vi "DeMux16x16.vi"(1 "Data":bool[](array[boolean]), 2 "Select":bool[](array[boolean])) -> (0 "A":bool[][](array[boolean]))   [LabVIEW 2012]
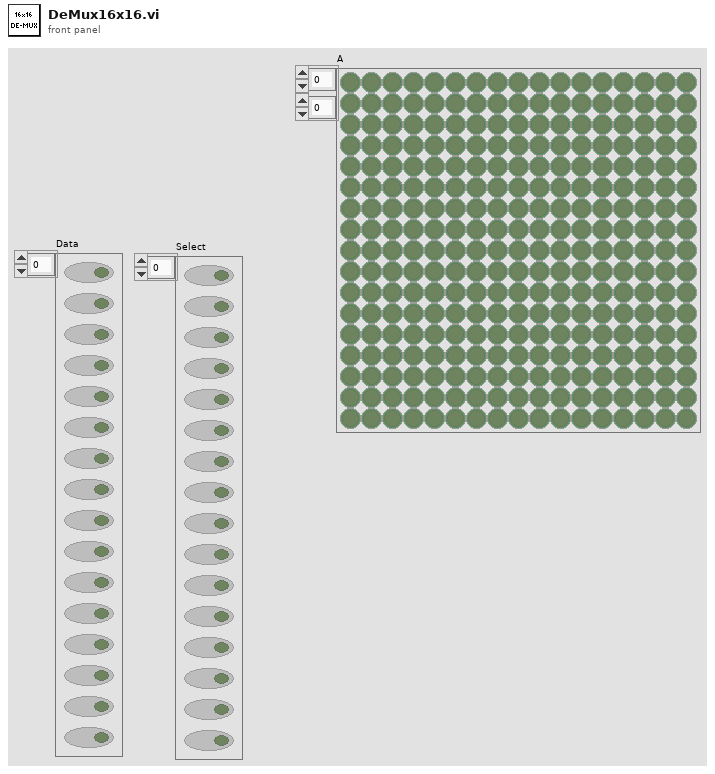
[diagram p1: front panel]
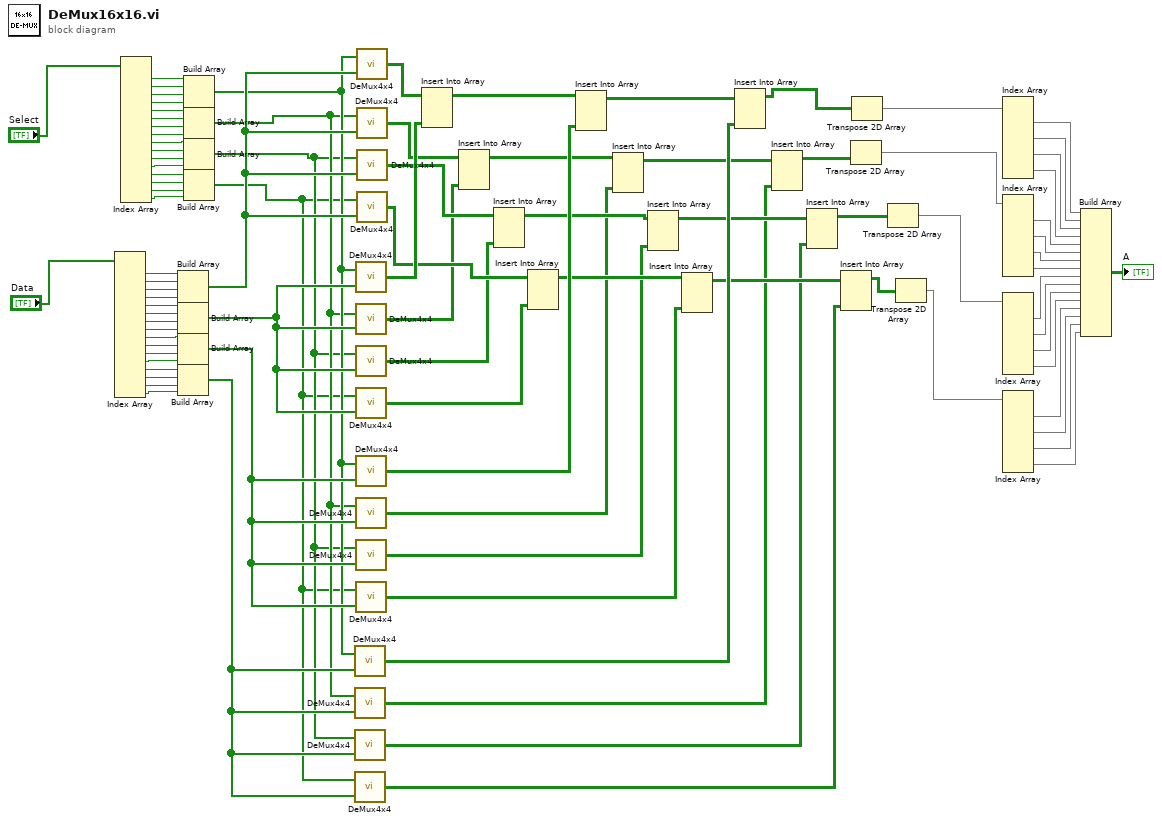
[diagram p0: block diagram]
diagram:
  n1 = Index Array(array="Data") -> (element #1=w59:bool, element #2=w60:bool, element #3=w61:bool, element #4=w62:bool, element #5=w63:bool, element #6=w64:bool, element #7=w65:bool, element #8=w66:bool, element #9=w67:bool, element #10=w68:bool, element #11=w69:bool, element #12=w70:bool, element #13=w71:bool, element #14=w72:bool, element #15=w73:bool, element #16=w74:bool)  [unwired: 16 in]
  n2 = Index Array(array="Select") -> (element #1=w91:bool, element #2=w90:bool, element #3=w89:bool, element #4=w88:bool, element #5=w87:bool, element #6=w86:bool, element #7=w85:bool, element #8=w84:bool, element #9=w83:bool, element #10=w82:bool, element #11=w81:bool, element #12=w80:bool, element #13=w79:bool, element #14=w78:bool, element #15=w77:bool, element #16=w76:bool)  [unwired: 16 in]
  n3 = Build Array(w59, w60, w61, w62) -> (w57:bool[])
  n4 = Build Array(w63, w64, w65, w66) -> (w56:bool[])
  n5 = Build Array(w67, w68, w69, w70) -> (w55:bool[])
  n6 = Build Array(w71, w72, w73, w74) -> (w54:bool[])
  n7 = Build Array(w91, w90, w89, w88) -> (w53:bool[])
  n8 = Build Array(w87, w86, w85, w84) -> (w52:bool[])
  n9 = Build Array(w83, w82, w81, w80) -> (w51:bool[])
  n10 = Build Array(w79, w78, w77, w76) -> (w50:bool[])
  n11 = call "DeMux4x4.vi"("Data"=w54, "Select"=w53) -> ("A"=w44:bool[][])
  n12 = call "DeMux4x4.vi"("Data"=w54, "Select"=w52) -> ("A"=w32:bool[][])
  n13 = call "DeMux4x4.vi"("Data"=w54, "Select"=w51) -> ("A"=w29:bool[][])
  n14 = call "DeMux4x4.vi"("Data"=w54, "Select"=w50) -> ("A"=w26:bool[][])
  n15 = call "DeMux4x4.vi"("Data"=w56, "Select"=w53) -> ("A"=w46:bool[][])
  n16 = call "DeMux4x4.vi"("Data"=w56, "Select"=w52) -> ("A"=w34:bool[][])
  n17 = call "DeMux4x4.vi"("Data"=w56, "Select"=w51) -> ("A"=w31:bool[][])
  n18 = call "DeMux4x4.vi"("Data"=w56, "Select"=w50) -> ("A"=w28:bool[][])
  n19 = call "DeMux4x4.vi"("Data"=w55, "Select"=w53) -> ("A"=w45:bool[][])
  n20 = call "DeMux4x4.vi"("Data"=w55, "Select"=w52) -> ("A"=w33:bool[][])
  n21 = call "DeMux4x4.vi"("Data"=w55, "Select"=w51) -> ("A"=w30:bool[][])
  n22 = call "DeMux4x4.vi"("Data"=w55, "Select"=w50) -> ("A"=w27:bool[][])
  n23 = call "DeMux4x4.vi"("Data"=w57, "Select"=w53) -> ("A"=w49:bool[][])
  n24 = call "DeMux4x4.vi"("Data"=w57, "Select"=w52) -> ("A"=w43:bool[][])
  n25 = call "DeMux4x4.vi"("Data"=w57, "Select"=w51) -> ("A"=w40:bool[][])
  n26 = call "DeMux4x4.vi"("Data"=w57, "Select"=w50) -> ("A"=w37:bool[][])
  n27 = Insert Into Array(array=w49, new element=w46) -> (w48:bool[][])  [unwired: 2 in]
  n28 = Insert Into Array(array=w43, new element=w34) -> (w42:bool[][])  [unwired: 2 in]
  n29 = Insert Into Array(array=w40, new element=w31) -> (w39:bool[][])  [unwired: 2 in]
  n30 = Insert Into Array(array=w37, new element=w28) -> (w36:bool[][])  [unwired: 2 in]
  n31 = Insert Into Array(array=w48, new element=w45) -> (w47:bool[][])  [unwired: 2 in]
  n32 = Insert Into Array(array=w42, new element=w33) -> (w41:bool[][])  [unwired: 2 in]
  n33 = Insert Into Array(array=w39, new element=w30) -> (w38:bool[][])  [unwired: 2 in]
  n34 = Insert Into Array(array=w36, new element=w27) -> (w35:bool[][])  [unwired: 2 in]
  n35 = Insert Into Array(array=w47, new element=w44) -> (w22:bool[][])  [unwired: 2 in]
  n36 = Insert Into Array(array=w41, new element=w32) -> (w25:bool[][])  [unwired: 2 in]
  n37 = Insert Into Array(array=w38, new element=w29) -> (w24:bool[][])  [unwired: 2 in]
  n38 = Insert Into Array(array=w35, new element=w26) -> (w23:bool[][])  [unwired: 2 in]
  n39 = Transpose 2D Array(2D array=w25) -> (transposed array=w20:bool[][])
  n40 = Transpose 2D Array(2D array=w22) -> (transposed array=w21:bool[][])
  n41 = Transpose 2D Array(2D array=w24) -> (transposed array=w19:bool[][])
  n42 = Transpose 2D Array(2D array=w23) -> (transposed array=w18:bool[][])
  n43 = Index Array(array=w21) -> (element #1=w17:bool[], element #2=w16:bool[], element #3=w15:bool[], element #4=w14:bool[])  [unwired: 8 in]
  n44 = Index Array(array=w20) -> (element #1=w13:bool[], element #2=w12:bool[], element #3=w11:bool[], element #4=w10:bool[])  [unwired: 8 in]
  n45 = Index Array(array=w19) -> (element #1=w9:bool[], element #2=w8:bool[], element #3=w7:bool[], element #4=w6:bool[])  [unwired: 8 in]
  n46 = Index Array(array=w18) -> (element #1=w5:bool[], element #2=w4:bool[], element #3=w3:bool[], element #4=w2:bool[])  [unwired: 8 in]
  n47 = Build Array(w17, w16, w15, w14, w13, w12, w11, w10, w9, w8, w7, w6, w5, w4, w3, w2) -> (→"A":bool[][])
